vi "Set Measurement Number.vi"(8 "error in (no error)":errorcluster, 11 "MCCW ACLR in":refnum<class "MCCW ACLR.lvclass">) -> (0 "error out":errorcluster, 1 "Parameter":cluster{"Name":string, "Value":string}, 2 "Last Carrier?":bool, 3 "MCCW ACLR out":refnum<class "MCCW ACLR.lvclass">)   [LabVIEW 2020, in "MCCW ACLR.lvclass"]
uses:
  MCCW ACLR.lvclass
  MCCW ACLR.lvclass/MCCW ACLR.ctl
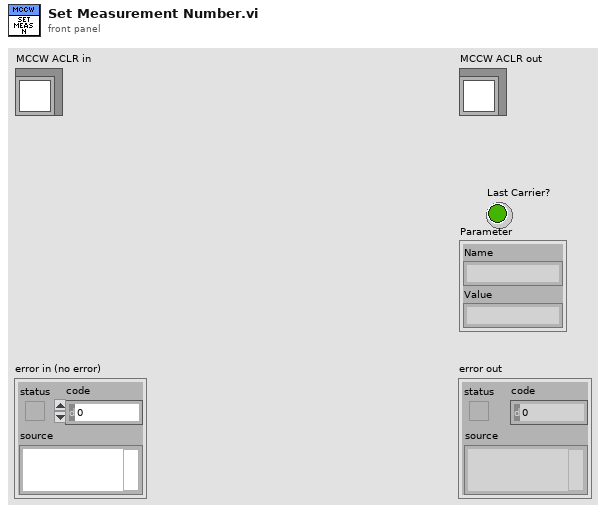
[diagram p1: front panel]
types:
  T1 = cluster{"Number of Measurements":u32, "Current Measurement":u32, "Last":bool}
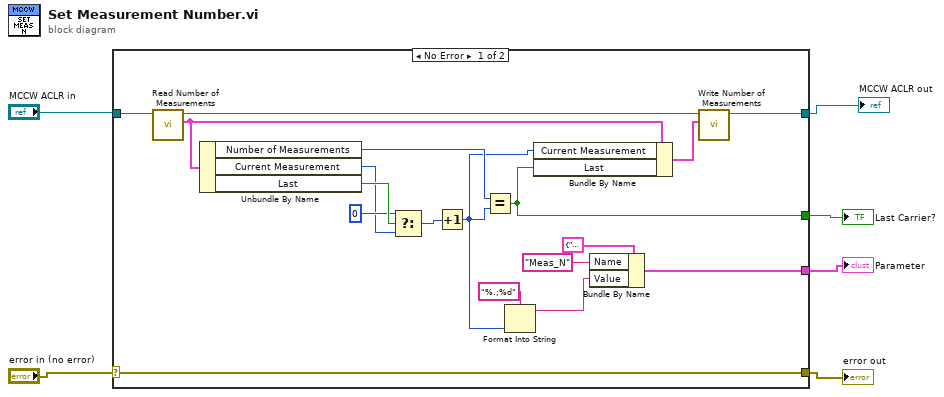
[diagram p0: block diagram]
diagram:
  n1 = case shown="No Error" "error in (no error)" {
    selector: "error in (no error)" -> [w17 w26]
    tunnel: [w17 w26] -> w5
    tunnel: [w18 w25] -> w3
    tunnel: "MCCW ACLR in" -> [w16 w25]
    tunnel: [w9 _] -> w2
    tunnel: [w19 _] -> w1
    frame No Error {
      n2 = call "Read Number of Measurements.vi"("MCCW ACLR in"=w16) -> ("Number of Measurements"=w10:T1, "MCCW ACLR out"=w24:refnum<class "MCCW ACLR.lvclass">)  [unwired: 9 in]
      n3 = Unbundle By Name(w10) -> ("Number of Measurements"=w15:u32, "Current Measurement"=w12:u32, "Last"=w14:bool)
      n4 = Select(t=u32 0, s=w14, f=w12) -> (s? t:f=w11:u32)
      n5 = Increment(x=w11) -> (x+1=w8:u32)
      n6 = Equal?(x=w15, y=w8) -> (x = y?=w9:bool)
      n7 = Format Into String(format string="%.;%d", w8) -> (resulting string=w20:string)  [unwired: 2 in, 1 out]
      n8 = Bundle By Name(cluster=w10, "Current Measurement"=w8, "Last"=w9) -> (w7:T1)
      n9 = Bundle By Name(cluster=cluster{"Name":string, "Value":string} {"Name"="", "Value"=""} ("Change"), "Name"="Meas_N", "Value"=w20) -> (w19:cluster{"Name":string, "Value":string})
      n10 = call "Write Number of Measurements.vi"("Number of Measurements"=w7, "MCCW ACLR in"=w24) -> ("MCCW ACLR out"=w18:refnum<class "MCCW ACLR.lvclass">)  [unwired: 9 in]
    }
    frame Error {
    }
  }
  "error out" <- w5
  "MCCW ACLR out" <- w3
  "Last Carrier?" <- w2
  "Parameter" <- w1
